vi "BaseplateCenterFinder.vi"() -> ()   [LabVIEW 2019]
uses:
  <vilib>/userDefined/High Color/IMAQdx.ctl
  <vilib>/Analysis/coordinate.llb/2D Cartesian Coordinate Rotation (Scalar).vi
  <vilib>/Analysis/baseanly.llb/Mean (DBL).vi
  Other Models/2010/Motion/AbortSingle.vi
  <vilib>/Analysis/NI_AALPro.lvlib
  <vilib>/vision/NI_Vision_Development_Module.lvlib
  <vilib>/Analysis/NI_AALBase.lvlib
panel:
  out "FileUsedForFiducials":string
  in  "Position":enum16{"1", "2"}(ring)
  in  "Zone":enum16{"ZoneA", "ZoneB", "ZoneC", "ZoneD"}(ring)
  in  "InitialStepSize":dbl=0.05
  in  "AbortAutoFocus":bool
  in  "AutoFocus":bool=TRUE
  out "UsedCoordinates 2":string
  out "UsedCoordinates":string
  in  "StopJoyStick":bool
  in  "VisibilityInCamera":enum16{"JoyStick", "ClickToMove", "AllVisible"}(ring)
  out "CameraGcode":string
  out "Output XYZU":string
  out "error out":errorcluster
  out "TempCoordinates":string
  in  "AdjustCamera":T1={"+Y"=FALSE, "-Z"=FALSE, "Done"=FALSE, "+Z"=FALSE, "-Y"=FALSE, "-X"=FALSE, "+X"=FALSE, "MoveXYBy(mm)"=0.25, "MoveZBy(mm)"=0.1} {"MoveZBy(mm)" format="%#_13g"}
  out "Image":T2(plugin-control)
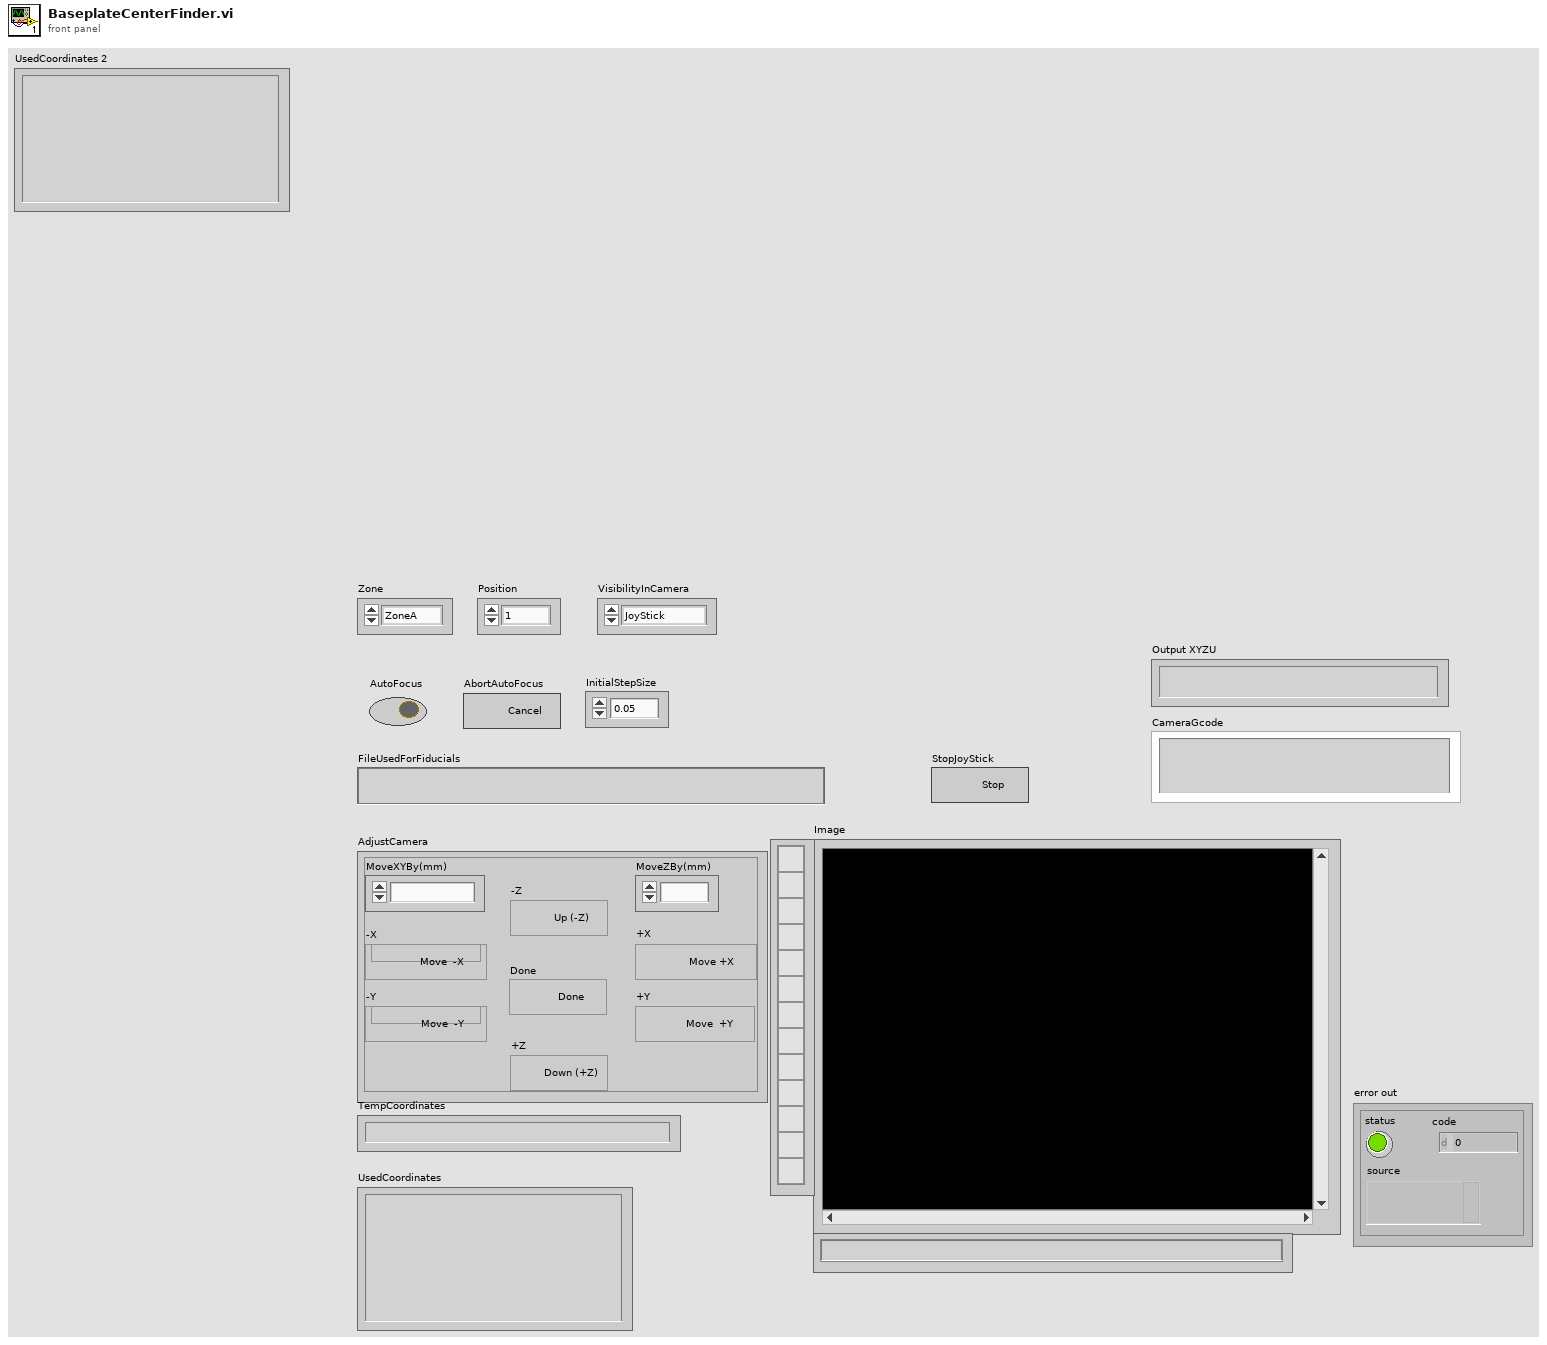
[diagram p1: front panel]
types:
  T1 = cluster{"+Y":bool, "-Z":bool, "Done":bool, "+Z":bool, "-Y":bool, "-X":bool, "+X":bool, "MoveXYBy(mm)":dbl, "MoveZBy(mm)":dbl}
  T2 = typedef "IMAQ Image.ctl" = refnum<image>
  T3 = typedef "IMAQdx.ctl" = refnum<k21>
  T4 = enum16{"Convolution", "Differentiation", "Gradient", "Prewitt", "Roberts", "Sigma", "Sobel"}
  T5 = typedef "IMAQ Point" = cluster{"X":sgl, "Y":sgl}
  T6 = cluster{"Point 1":cluster{"X":sgl, "Y":sgl}, "Point 2":cluster{"X":sgl, "Y":sgl}}
  T7 = enum16{"Left Button", "Center Button", "Right Button", "Window Close"}
  T8 = enum16{"open", "replace", "create", "open or create", "replace or create", "replace or create with confirmation"}
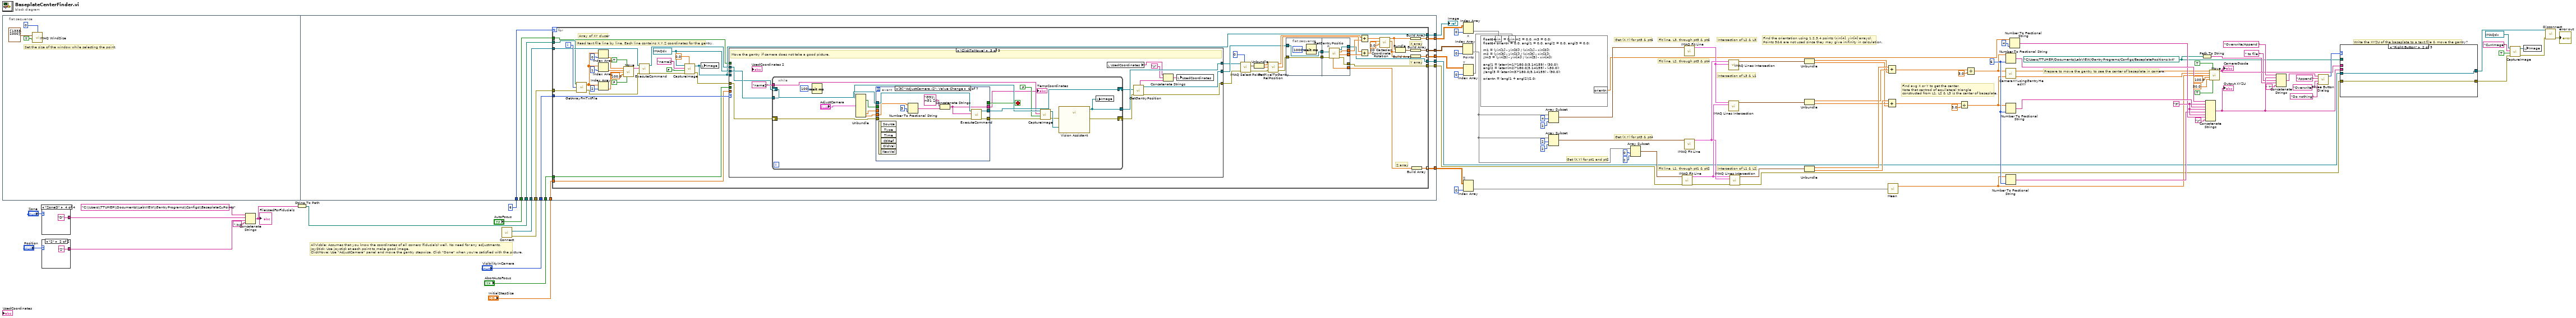
[diagram p0: block diagram]
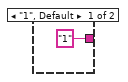
[diagram p2: hidden frame]
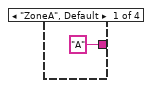
[diagram p3: hidden frame]
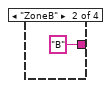
[diagram p4: hidden frame]
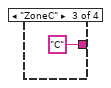
[diagram p5: hidden frame]
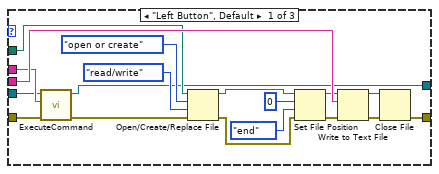
[diagram p6: hidden frame]
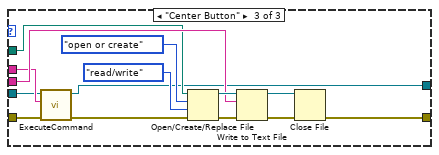
[diagram p7: hidden frame]
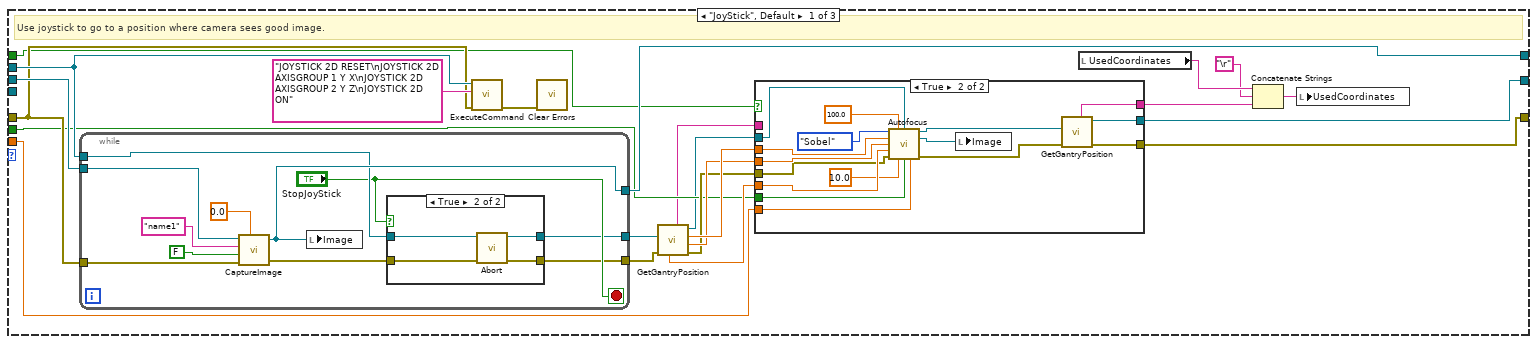
[diagram p8: hidden frame]
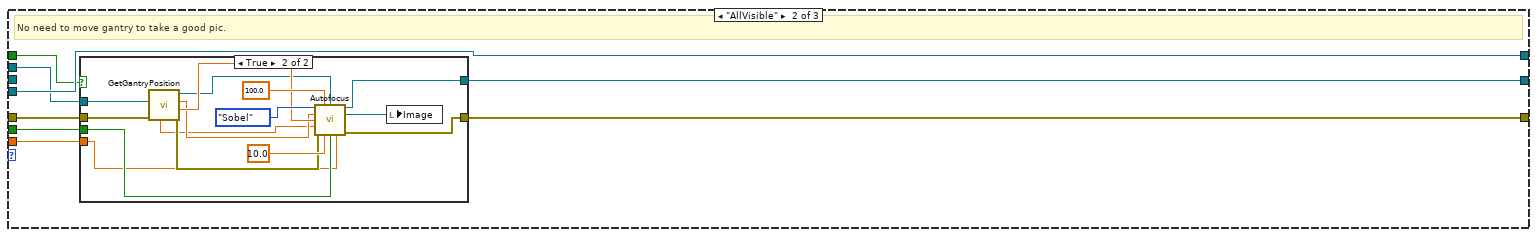
[diagram p11: hidden frame]
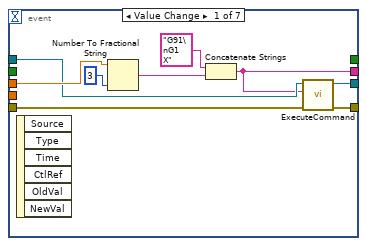
[diagram p13: hidden frame]
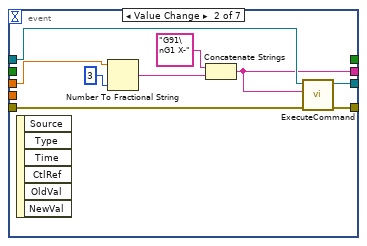
[diagram p14: hidden frame]
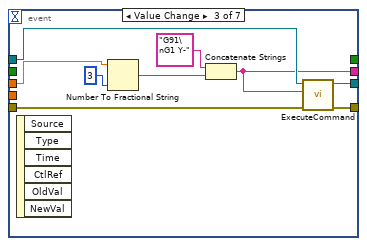
[diagram p15: hidden frame]
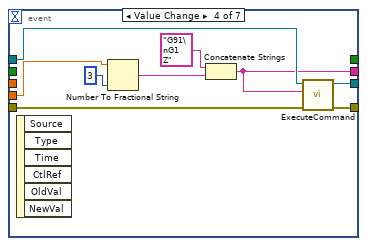
[diagram p16: hidden frame]
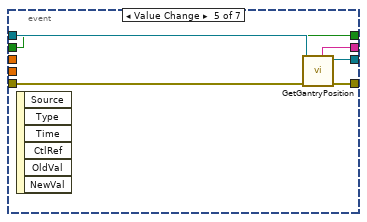
[diagram p17: hidden frame]
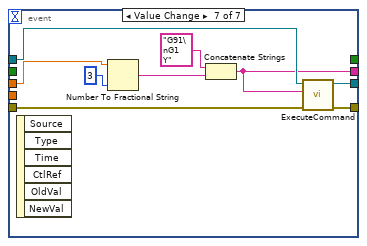
[diagram p18: hidden frame]
diagram:
  w18 = path "C:/Users/TTUHEP/Documents/LabVIEW/GantryPrograms/Configs/BaseplatePositions.txt" ("OutFile")
  w50 = "\t"
  w47 = i16 6 ("width (-)")
  # "Write the XYZU of the baseplate to a text file & move the gantry?"
  # "Prepare to move the gantry to see the center of baseplate in camera."
  # "Find avg X or Y to get the center. \nNote that centrod of equilateral triangle\nconstructed from L1, L2 & L3 is the center of baseplate."
  # "Intersection of L3 & L1"
  # "Intersection of L1 & L2."
  # "Fit line, L1, through pt1 & pt2"
  # "Intersection of L2 & L3"
  # "Fit line, L3, through pt5 & pt6"
  # "Fit line, L2, through pt3 & pt4"
  # "Get (X,Y) for pt3 & pt4"
  # "Get (X,Y) for pt5 & pt6"
  # "Get (X,Y) for pt1 and pt2"
  # "Find the orientation using 1,2,3,4 points (xin[4], yin[4] arrays).\nPoints 5&6 are not used since they may give inifinity in calculation."
  # "AllVisble: Assumes that you know the coordinates of all corners (fiducials) well. No need for any adjustments.\nJoyStick: Use joystick at each point to make good image.\nClickMove: Use \"AdjustCamera\" panel and move the gantry stepwise. Click \"Done\" when you're satisfied with the picture."
  n1 = flat-sequence {
    tunnel: 6 -> [w113]
    tunnel: w94 -> [w112]
    tunnel: w93 -> [w111]
    tunnel: w4 -> [w110]
    tunnel: [w109] -> w92
    tunnel: [w108] -> w90
    tunnel: [w107] -> w87
    tunnel: [w106] -> w86
    tunnel: [w105] -> w85
    tunnel: [w104] -> w70
    tunnel: [w103] -> w20
    tunnel: "VisibilityInCamera" -> [w102]
    tunnel: "AbortAutoFocus" -> [w101]
    tunnel: "AutoFocus" -> [w100]
    tunnel: "InitialStepSize" -> [w99]
    frame #0 {
      # "Set the size of the window while selecting the point."
      n2 = call "IMAQ WindSize"("Scrollbars? (N)"=TRUE, "Width & Height"=cluster{"Width":i32, "Height":i32} {"Width"=1333, "Height"=1000}, "Window Number"=0) -> ()  [unwired: 3 in, 3 out]
    }
    frame #1 {
      n3 = for {
        N: w113 -> [_]
        tunnel: w112 -> [w129]
        tunnel: w111 -> [w158]
        tunnel: [w117] -> w109
        tunnel: w110 -> [w130]
        tunnel: [w127] -> w108 mode=indexing
        tunnel: [w126] -> w107 mode=indexing
        tunnel: [w125] -> w106 mode=indexing
        tunnel: [w121] -> w105 mode=indexing
        tunnel: [w120] -> w104
        tunnel: [w119] -> w103
        tunnel: w102 -> [w118]
        tunnel: w101 -> [w116]
        tunnel: w100 -> [w115]
        tunnel: w99 -> [w114]
        i -> [w159]
        w153 = T3 "cam0" ("Camera")
        # "Array of XY cluser"
        # "Z array"
        # "Y array"
        # "X array"
        # "Read text file line by line. Each line contains X,Y,Z coordinates for the gantry."
        n4 = call "GetArrayFmTxtFile.vi"("error in"=w129, "LineNo."=w159, "TextFile"=w130) -> ("error out"=w128:errorcluster, "Array"=w166:dbl[])
        n5 = Index Array(array=w166, index=0) -> (element=w161:dbl)
        n6 = Index Array(array=w166, index=1) -> (element=w160:dbl)
        n7 = Index Array(array=w166, index=2) -> (element=w162:dbl)
        n8 = call "Move.vi"("X"=w161, "Absolute"=TRUE, "Y"=w160, "Z"=w162, "SpeedXY (mm/s)"=100.0, "Move Z first"=FALSE) -> ("Position Gcode"=w157:string)  [unwired: 9 in]
        n9 = call "ExecuteCommand.vi"("error in (no error)"=w128, "Command Code"=w157, "controller in"=w158) -> ("error out"=w155:errorcluster, "controller out"=w152:refnum<k24>)  [unwired: 6 in, 1 out]
        n10 = call "CaptureImage.vi"("Camera"=w153, "Rotate (degrees)"=sgl 0.0, "ImageName"="name1", "Draw50MicroCircleAtCenter"=FALSE, "error in (no error)"=w155) -> ("Image"=w117:T2, "error out"=w151:errorcluster)  [unwired: 2 in]
        n11 = local write "Image"(w117) -> ()
        n12 = case shown="\"ClickToMove\"" w118 {
          tunnel: w153 -> [w201 _ w275]
          tunnel: w152 -> [w199 w242 w274]
          tunnel: w151 -> [w197 w243 w273]
          tunnel: [w200 w246 w272] -> w134
          tunnel: [w183 w245 w264] -> w136
          tunnel: [w184 w244 w266] -> w135
          tunnel: w117 -> [_ w246 _]
          tunnel: w116 -> [w187 w240 _]
          tunnel: w115 -> [w181 w241 _]
          tunnel: w114 -> [w180 w239 _]
          frame "JoyStick", Default {
            # "Use joystick to go to a position where camera sees good image."
            n13 = while {
              tunnel: w201 -> [w231]
              tunnel: [w228] -> w200
              tunnel: w199 -> [w227]
              tunnel: [w224] -> w195
              tunnel: [w223] -> w196
              tunnel: w197 -> [w222]
              stop <- "StopJoyStick" stop-if-true
              n14 = call "CaptureImage.vi"("Camera"=w231, "Rotate (degrees)"=sgl 0.0, "ImageName"="name1", "Draw50MicroCircleAtCenter"=FALSE, "error in (no error)"=w222) -> ("Image"=w228:T2, "error out"=w225:errorcluster)  [unwired: 2 in]
              n15 = local write "Image"(w228) -> ()
              n16 = case shown="True" "StopJoyStick" {
                tunnel: w227 -> [w234 w238]
                tunnel: w225 -> [w233 w237]
                tunnel: [w233 w236] -> w224
                tunnel: [w234 w235] -> w223
                frame False {
                }
                frame True {
                  n17 = call-poly "Abort.vi"("error in (no error)"=w237, "controller in"=w238) -> ("error out"=w236:errorcluster, "controller out"=w235:refnum<k24>)  [unwired: 8 in]
                }
              }
            }
            n18 = call "ExecuteCommand.vi"("error in (no error)"=w197, "Command Code"="JOYSTICK 2D RESET\nJOYSTICK 2D AXISGROUP 1 Y X\nJOYSTICK 2D AXISGROUP 2 Y Z\nJOYSTICK 2D ON", "controller in"=w199) -> ("error out"=w198:errorcluster)  [unwired: 6 in, 2 out]
            n19 = call <vilib>:"Clear Errors.vi"("error in (no error)"=w198) -> ()  [unwired: 5 in, 2 out]
            n20 = call "GetGantryPosition.vi"("error in (no error)"=w195, "Controller In"=w196) -> ("error out"=w188:errorcluster, "Position Y"=w190:dbl, "Position X"=w191:dbl, "controller out"=w186:refnum<k24>, "Position_XYZ"=w182:string, "Position Z"=w189:dbl)  [unwired: 3 in, 1 out]
            n21 = case shown="True" w181 {
              tunnel: w191 -> [_ w220]
              tunnel: w190 -> [_ w219]
              tunnel: w189 -> [_ w218]
              tunnel: w188 -> [w205 w217]
              tunnel: w187 -> [_ w215]
              tunnel: w186 -> [w203 w214]
              tunnel: [w204 w210] -> w185
              tunnel: [w205 w209] -> w184
              tunnel: [w203 w208] -> w183
              tunnel: w182 -> [w204 _]
              tunnel: w180 -> [_ w206]
              frame False {
              }
              frame True {
                n22 = call "Autofocus.vi"("Filter Type"=T4."Sobel", "SpeedXY (mm/s)"=100.0, "controller in"=w214, "X"=w220, "Y"=w219, "Z"=w218, "error in (no error)"=w217, "SpeedZ (mm/s)"=10.0, "AbortAutoFocus"=w215, "InitialStepSize"=w206) -> ("controller out"=w212:refnum<k24>, "Image"=w207:T2, "error out"=w211:errorcluster)  [unwired: 2 in, 1 out]
                n23 = local write "Image"(w207) -> ()
                n24 = call "GetGantryPosition.vi"("error in (no error)"=w211, "Controller In"=w212) -> ("error out"=w209:errorcluster, "controller out"=w208:refnum<k24>, "Position_XYZ"=w210:string)  [unwired: 3 in, 4 out]
              }
            }
            n25 = local read "UsedCoordinates"() -> (w193:string)
            n26 = Concatenate Strings(w193, "\r", w185) -> (w194:string)
            n27 = local write "UsedCoordinates"(w194) -> ()
          }
          frame "AllVisible" {
            # "No need to move gantry to take a good pic."
            n28 = case shown="True" w241 {
              tunnel: w240 -> [_ w261]
              tunnel: [w248 w258] -> w244
              tunnel: [w247 w259] -> w245
              tunnel: w243 -> [w248 w257]
              tunnel: w242 -> [w247 w256]
              tunnel: w239 -> [_ w249]
              frame False {
              }
              frame True {
                n29 = call "GetGantryPosition.vi"("error in (no error)"=w257, "Controller In"=w256) -> ("error out"=w255:errorcluster, "Position Y"=w254:dbl, "Position X"=w253:dbl, "controller out"=w252:refnum<k24>, "Position Z"=w251:dbl)  [unwired: 3 in, 2 out]
                n30 = call "Autofocus.vi"("Filter Type"=T4."Sobel", "SpeedXY (mm/s)"=100.0, "controller in"=w252, "X"=w253, "Y"=w254, "Z"=w251, "error in (no error)"=w255, "SpeedZ (mm/s)"=10.0, "AbortAutoFocus"=w261, "InitialStepSize"=w249) -> ("controller out"=w259:refnum<k24>, "Image"=w250:T2, "error out"=w258:errorcluster)  [unwired: 2 in, 1 out]
                n31 = local write "Image"(w250) -> ()
              }
            }
          }
          frame "ClickToMove" {
            # "Move the gantry if camera does not take a good picture."
            n32 = while {
              shift-right: [w286] -> w267
              shift-left: w273 -> [w294]
              shift-right: [w292] -> w265
              shift-left: w274 -> [w293]
              tunnel: "name2" ("ImageName") -> [w288]
              tunnel: w275 -> [w289]
              tunnel: [w279] -> w272
              stop <- w291 stop-if-true
              n33 = Wait (ms)(milliseconds to wait=u32 100) -> ()  [unwired: 1 out]
              n34 = Unbundle("AdjustCamera") -> ("Done"=w282:bool, "MoveXYBy(mm)"=w280:dbl, "MoveZBy(mm)"=w281:dbl)  [unwired: 6 out]
              n35 = event shown="[5] \"AdjustCamera.-Z\": Value Change" {
                selector: _ -> [_ _ _ _ _ _ _]
                dyn-events: _ -> [_ _ _ _ _ _ _]
                timeout: _ -> [_ _ _ _ _ _ _]
                tunnel: w280 -> [w300 w304 w313 _ _ _ w346]
                tunnel: w294 -> [w299 w308 w317 w326 w335 w341 w350]
                tunnel: [w298 w307 w316 w323 w332 w340 w349] -> w287
                tunnel: w293 -> [w297 w309 w318 w327 w336 w342 w351]
                tunnel: [w296 w306 w315 w324 w334 w339 w348] -> w292
                tunnel: [w295 w305 w314 w325 w333 w338 w347] -> w277
                tunnel: [_ _ _ _ w331 _ _] -> w291
                tunnel: w281 -> [_ _ _ w322 _ w337 _]
                tunnel: w282 -> [_ _ _ _ w331 _ _]
                event "AdjustCamera.+X": Value Change {
                  n36 = event-data() -> ()  [unwired: 1 in, 6 out]
                  n37 = Number To Fractional String(number=w300, precision (6)=3) -> (F-format string=w303:string)  [unwired: 2 in]
                  n38 = Concatenate Strings("G91\nG1 X", w303) -> (w295:string)
                  n39 = call "ExecuteCommand.vi"("error in (no error)"=w299, "Command Code"=w295, "controller in"=w297) -> ("error out"=w298:errorcluster, "controller out"=w296:refnum<k24>)  [unwired: 6 in, 1 out]
                }
                event "AdjustCamera.-X": Value Change {
                  n40 = event-data() -> ()  [unwired: 1 in, 6 out]
                  n41 = Number To Fractional String(number=w304, precision (6)=3) -> (F-format string=w312:string)  [unwired: 2 in]
                  n42 = Concatenate Strings("G91\nG1 X-", w312) -> (w305:string)
                  n43 = call "ExecuteCommand.vi"("error in (no error)"=w308, "Command Code"=w305, "controller in"=w309) -> ("error out"=w307:errorcluster, "controller out"=w306:refnum<k24>)  [unwired: 6 in, 1 out]
                }
                event "AdjustCamera.-Y": Value Change {
                  n44 = event-data() -> ()  [unwired: 1 in, 6 out]
                  n45 = Number To Fractional String(number=w313, precision (6)=3) -> (F-format string=w321:string)  [unwired: 2 in]
                  n46 = Concatenate Strings("G91\nG1 Y-", w321) -> (w314:string)
                  n47 = call "ExecuteCommand.vi"("error in (no error)"=w317, "Command Code"=w314, "controller in"=w318) -> ("error out"=w316:errorcluster, "controller out"=w315:refnum<k24>)  [unwired: 6 in, 1 out]
                }
                event "AdjustCamera.+Z": Value Change {
                  n48 = event-data() -> ()  [unwired: 1 in, 6 out]
                  n49 = Number To Fractional String(number=w322, precision (6)=3) -> (F-format string=w330:string)  [unwired: 2 in]
                  n50 = Concatenate Strings("G91\nG1 Z", w330) -> (w325:string)
                  n51 = call "ExecuteCommand.vi"("error in (no error)"=w326, "Command Code"=w325, "controller in"=w327) -> ("error out"=w323:errorcluster, "controller out"=w324:refnum<k24>)  [unwired: 6 in, 1 out]
                }
                event "AdjustCamera.Done": Value Change {
                  n52 = event-data() -> ()  [unwired: 1 in, 6 out]
                  n53 = call "GetGantryPosition.vi"("error in (no error)"=w335, "Controller In"=w336) -> ("error out"=w332:errorcluster, "controller out"=w334:refnum<k24>, "Position_XYZ"=w333:string)  [unwired: 3 in, 4 out]
                }
                event "AdjustCamera.-Z": Value Change {
                  n54 = event-data() -> ()  [unwired: 1 in, 6 out]
                  n55 = Number To Fractional String(number=w337, precision (6)=3) -> (F-format string=w345:string)  [unwired: 2 in]
                  n56 = Concatenate Strings("G91\nG1 Z-", w345) -> (w338:string)
                  n57 = call "ExecuteCommand.vi"("error in (no error)"=w341, "Command Code"=w338, "controller in"=w342) -> ("error out"=w340:errorcluster, "controller out"=w339:refnum<k24>)  [unwired: 6 in, 1 out]
                }
                event "AdjustCamera.+Y": Value Change {
                  n58 = event-data() -> ()  [unwired: 1 in, 6 out]
                  n59 = Number To Fractional String(number=w346, precision (6)=3) -> (F-format string=w354:string)  [unwired: 2 in]
                  n60 = Concatenate Strings("G91\nG1 Y", w354) -> (w347:string)
                  n61 = call "ExecuteCommand.vi"("error in (no error)"=w350, "Command Code"=w347, "controller in"=w351) -> ("error out"=w349:errorcluster, "controller out"=w348:refnum<k24>)  [unwired: 6 in, 1 out]
                }
              }
              "TempCoordinates" <- w277
              n62 = call "CaptureImage.vi"("Camera"=w289, "ImageName"=w288, "Draw50MicroCircleAtCenter"=FALSE, "error in (no error)"=w287) -> ("Image"=w285:T2, "error out"=w284:errorcluster)  [unwired: 3 in]
              n63 = call "Vision Assistant"("Image In"=w285, "error in"=w284) -> ("Image Out"=w279:T2, "error out"=w286:errorcluster)  [unwired: 24 in]
              n64 = local write "Image"(w279) -> ()
            }
            n65 = local read "UsedCoordinates"() -> (w270:string)
            n66 = call "GetGantryPosition.vi"("error in (no error)"=w267, "Controller In"=w265) -> ("error out"=w266:errorcluster, "controller out"=w264:refnum<k24>, "Position_XYZ"=w268:string)  [unwired: 3 in, 4 out]
            n67 = Concatenate Strings(w270, "\r", w268) -> (w271:string)
            n68 = local write "UsedCoordinates"(w271) -> ()
          }
        }
        n69 = call "IMAQ Select Point"("Window Number (0...15)"=0, "error in (no error)"=w135, "Image In"=w134) -> ("error out"=w143:errorcluster, "Point"=w146:T5)  [unwired: 5 in, 2 out]
        n70 = Unbundle(w146) -> ("X"=w145:sgl, "Y"=w144:sgl)
        n71 = call "GetPixelToGantryRelPosition.vi"("error in (no error)"=w143, "PixelY"=w144, "PixelX"=w145) -> ("error out"=w137:errorcluster, "YmmRelGH"=w141:dbl, "XmmRelGH"=w142:dbl)
        n72 = flat-sequence {
          tunnel: w137 -> [w171]
          tunnel: [w171] -> w149
          tunnel: w136 -> [w170]
          tunnel: [w170] -> w148
          tunnel: [w179] -> w120
          tunnel: [w178] -> w140
          tunnel: [w177] -> w139
          tunnel: [w176] -> w119
          tunnel: [w175] -> w138
          tunnel: w149 -> [w174]
          tunnel: w148 -> [w173]
          frame #0 {
            n73 = Wait (ms)(milliseconds to wait=u32 1000) -> ()  [unwired: 1 out]
          }
          frame #1 {
            n74 = call "GetGantryPosition.vi"("error in (no error)"=w174, "Controller In"=w173) -> ("error out"=w179:errorcluster, "Position Y"=w178:dbl, "Position X"=w177:dbl, "controller out"=w176:refnum<k24>, "Position Z"=w175:dbl)  [unwired: 3 in, 2 out]
          }
        }
        n75 = Add(x=w142, y=w139) -> (x+y=w133:dbl)
        n76 = Add(x=w141, y=w140) -> (x+y=w132:dbl)
        n77 = call-poly <vilib>:"2D Cartesian Coordinate Rotation.vi"("theta"=0.0, "y"=w132, "x"=w133) -> ("y out"=w123:dbl, "x out"=w124:dbl)  [unwired: 6 in, 1 out]
        n78 = Bundle("x out"=w124, "y out"=w123) -> (w122:cluster{"x out":dbl, "y out":dbl})  [unwired: 1 in]
        n79 = Build Array(w122) -> (w121:cluster{"x out":dbl, "y out":dbl}[])
        n80 = Build Array(w124) -> (w127:dbl[])
        n81 = Build Array(w123) -> (w126:dbl[])
        n82 = Build Array(w138) -> (w125:dbl[])
      }
    }
  }
  n83 = case shown="\"ZoneD\"" "Zone" {
    tunnel: ["A" "B" "C" "D"] -> w7
    frame "ZoneA", Default {
    }
    frame "ZoneB" {
    }
    frame "ZoneC" {
    }
    frame "ZoneD" {
    }
  }
  n84 = case shown="\"2\"" "Position" {
    tunnel: ["1" "2"] -> w6
    frame "1", Default {
    }
    frame "2" {
    }
  }
  n85 = Concatenate Strings("C:\\Users\\TTUHEP\\Documents\\LabVIEW\\GantryPrograms\\Configs\\BaseplateCuPoints", w7, w6, ".txt" ("string")) -> (w5:string)
  "FileUsedForFiducials" <- w5
  n86 = String To Path(string=w5) -> (path=w4:path)
  n87 = call "Connect.vi"() -> ("error out"=w94:errorcluster, "controller"=w93:refnum<k24>)  [unwired: 10 in]
  n88 = Index Array "Points"(array=w85, index (col)=0 ("disabled index (col)")) -> (element=w74:cluster{"x out":dbl, "y out":dbl}[])  [unwired: 1 in]
  n89 = Index Array "X"(array=w90, index (col)=0 ("disabled index (col)")) -> (element=w54:dbl[])  [unwired: 1 in]
  n90 = Index Array "Y"(array=w87, index (col)=0 ("disabled index (col)")) -> (element=w53:dbl[])  [unwired: 1 in]
  n91 = Index Array "Z"(array=w86, index (col)=0 ("disabled index (col)")) -> (element=w55:dbl[])  [unwired: 1 in]
  n92 = formula code="float64 m1 = 0.0, m2 = 0.0, m3 = 0.0;\nfloat64 orientn = 0.0, angl1 = 0.0, angl2 = 0.0, angl3 = 0.0;\n\nm1 = (yin[1] - yin[0]) / (xin[1] - xin[0]);\nm2 = (yin[3] - yin[2]) / (xin[3] - xin[2]);\n//m3 = (yin[5] - yin[4]) / (xin[5] - xin[4]);\n\nangl1 = (atan(m1)*180.0/3.14159) - (30.0);\nangl2 = (atan(m2)*180.0/3.14159) - (-30.0);\n//angl3 = (atan(m3)*180.0/3.14159) - (90.0);\n\norientn = (angl1 + angl2)/2.0;"("xin"=w54, "yin"=w53) -> ("orientn"=w23:dbl)
  n93 = Array Subset(array=w74, index=4, length=2) -> (w75:cluster{"x out":dbl, "y out":dbl}[])
  n94 = Array Subset(array=w74, index=2, length=2) -> (w78:cluster{"x out":dbl, "y out":dbl}[])
  n95 = Array Subset(array=w74, index=0, length=2) -> (w81:cluster{"x out":dbl, "y out":dbl}[])
  n96 = call "IMAQ Fit Line"("error in (no error)"=w70, "Points"=w81) -> ("error out"=w69:errorcluster, "Line Segment"=w71:T6)  [unwired: 4 in, 4 out]
  n97 = call "IMAQ Fit Line"("Points"=w75) -> ("Line Segment"=w72:T6)  [unwired: 5 in, 5 out]
  n98 = call "IMAQ Fit Line"("Points"=w78) -> ("Line Segment"=w73:T6)  [unwired: 5 in, 5 out]
  n99 = call "IMAQ Lines Intersection"("Line 2"=w72, "Line 1"=w73) -> ("Intersection Point"=w56:cluster{"X":sgl, "Y":sgl})  [unwired: 7 in, 2 out]
  n100 = call "IMAQ Lines Intersection"("Line 2"=w71, "Line 1"=w72) -> ("Intersection Point"=w57:cluster{"X":sgl, "Y":sgl})  [unwired: 7 in, 2 out]
  n101 = call "IMAQ Lines Intersection"("error in (no error)"=w69, "Line 2"=w73, "Line 1"=w71) -> ("error out"=w22:errorcluster, "Intersection Point"=w58:cluster{"X":sgl, "Y":sgl})  [unwired: 6 in, 1 out]
  n102 = Unbundle(w56) -> ("X"=w66:sgl, "Y"=w59:sgl)
  n103 = Unbundle(w57) -> ("X"=w67:sgl, "Y"=w60:sgl)
  n104 = Unbundle(w58) -> ("X"=w68:sgl, "Y"=w61:sgl)
  n105 = call-poly <vilib>:"Mean.vi"("X"=w55) -> ("mean"=w24:dbl)  [unwired: 1 out]
  n106 = Compound Arithmetic op=ADD(w68, w67, w66) -> (w65:sgl)
  n107 = Compound Arithmetic op=ADD(w61, w60, w59) -> (w63:sgl)
  n108 = Divide(x=w63, y=sgl 3.0) -> (x/y=w25:sgl)
  n109 = Divide(x=w65, y=sgl 3.0) -> (x/y=w26:sgl)
  n110 = Number To Fractional String(number=w26, precision (6)=w47) -> (F-format string=w52:string)  [unwired: 2 in]
  n111 = call "CameraXYusingGantryHeadXY.vi"("GantryY"=w25, "GantryX"=w26) -> ("CamY"=w31:dbl, "CamX"=w32:dbl)
  n112 = Number To Fractional String(number=w25, precision (6)=w47) -> (F-format string=w51:string)  [unwired: 2 in]
  n113 = Number To Fractional String(number=w24, precision (6)=w47) -> (F-format string=w46:string)  [unwired: 2 in]
  n114 = Number To Fractional String(number=w23, precision (6)=i16 4 ("width (-)")) -> (F-format string=w48:string)  [unwired: 2 in]
  n115 = Path To String(path=w18) -> (string=w19:string)
  n116 = Concatenate Strings(w52, w50, w51, w50, w46, w50, w48, "\r") -> (w44:string)
  "Output XYZU" <- w44
  n117 = call "Move.vi"("X"=w32, "Absolute"=TRUE, "Y"=w31, "Z"=w24, "SpeedXY (mm/s)"=100.0, "SpeedZ (mm/s)"=50.0, "Move Z first"=TRUE) -> ("Position Gcode"=w30:string)  [unwired: 8 in]
  "CameraGcode" <- w30
  n118 = Concatenate Strings("Overwrite/Append ", w44, " to file ", w19, " ?" ("string")) -> (w41:string)
  n119 = call <vilib>:"Three Button Dialog.vi"("Right Button Text (\"Cancel\")"="Do nothing" ("Right Button Text (\"Cancel\")"), "Center Button Text (\"No\")"="Overwrite" ("Left Button Text (\"Yes\")"), "Left Button Text (\"Yes\")"="Append" ("Center Button Text (\"No\")"), "message"=w41) -> ("Which Button?"=w40:T7)  [unwired: 7 in]
  n120 = case shown="\"Right Button\"" w40 {
    tunnel: w44 -> [w374 _ w388]
    tunnel: w18 -> [w373 _ w387]
    tunnel: w22 -> [w372 w380 w386]
    tunnel: w30 -> [w371 _ w385]
    tunnel: w20 -> [w370 w379 w384]
    tunnel: [w361 w380 w381] -> w29
    tunnel: [w369 w379 w383] -> w28
    frame "Left Button", Default {
      n121 = call "ExecuteCommand.vi"("error in (no error)"=w372, "Command Code"=w371, "controller in"=w370) -> ("error out"=w362:errorcluster, "controller out"=w369:refnum<k24>)  [unwired: 6 in, 1 out]
      n122 = Open/Create/Replace File(file path (use dialog)=w373, error in=w362, operation (0:open)=T8."open or create", access (0:read/write)=enum16{"read/write", "read-only", "write-only"}."read/write") -> (refnum out=w366:refnum<file>, error out=w364:errorcluster)  [unwired: 2 in, 1 out]
      n123 = Set File Position(offset (in bytes) (0)=i64 0, refnum=w366, from (0:start)=enum16{"start", "end", "current"}."end", error in=w364) -> (refnum out=w365:refnum<file>, error out=w363:errorcluster)
      n124 = Write to Text File(file (use dialog)=w365, text=w374, error in=w363) -> (refnum out=w375:refnum<file>, error out=w376:errorcluster)  [unwired: 1 in, 1 out]
      n125 = Close File(refnum=w375, error in=w376) -> (error out=w361:errorcluster)  [unwired: 1 out]
    }
    frame "Right Button" {
    }
    frame "Center Button" {
      n126 = call "ExecuteCommand.vi"("error in (no error)"=w386, "Command Code"=w385, "controller in"=w384) -> ("error out"=w382:errorcluster, "controller out"=w383:refnum<k24>)  [unwired: 6 in, 1 out]
      n127 = Open/Create/Replace File(file path (use dialog)=w387, error in=w382, operation (0:open)=T8."open or create", access (0:read/write)=enum16{"read/write", "read-only", "write-only"}."read/write") -> (refnum out=w394:refnum<file>, error out=w391:errorcluster)  [unwired: 2 in, 1 out]
      n128 = Write to Text File(file (use dialog)=w394, text=w388, error in=w391) -> (refnum out=w389:refnum<file>, error out=w390:errorcluster)  [unwired: 1 in, 1 out]
      n129 = Close File(refnum=w389, error in=w390) -> (error out=w381:errorcluster)  [unwired: 1 out]
    }
  }
  n130 = call "CaptureImage.vi"("Camera"=T3 "cam0", "ImageName"="CurrImage", "Draw50MicroCircleAtCenter"=TRUE, "error in (no error)"=w29) -> ("Image"=w17:T2, "error out"=w35:errorcluster)  [unwired: 3 in]
  n131 = local write "Image"(w17) -> ()
  n132 = call "Disconnect.vi"("error in (no error)"=w35, "controller"=w28) -> ("error out"=→"error out":errorcluster)  [unwired: 9 in]
  "Image" <- w92
